vi "Create.vi"(8 "error in (no error)":errorcluster, 10 "Data Count":i32) -> (0 "error out":errorcluster, 3 "Data Count Msg out":refnum<class "Data Count Msg.lvclass">)   [LabVIEW 2022 SP3, in "Scratchpad.lvlib" / "Test 1.lvlib" / "Data Count Msg.lvclass"]
uses:
  Data Count Msg.lvclass
  Data Count Msg.lvclass/Data Count Msg.ctl
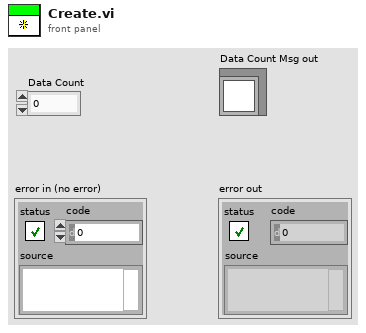
[diagram p1: front panel]
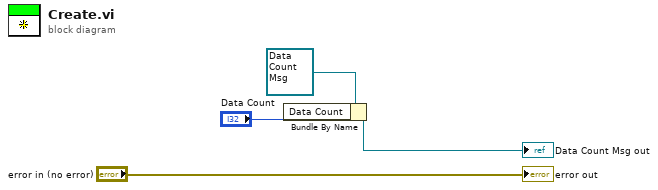
[diagram p0: block diagram]
diagram:
  n1 = Bundle By Name(cluster=refnum<class "Data Count Msg.lvclass"> refnum ("Data Count Msg in"), "Data Count"="Data Count") -> (→"Data Count Msg out":refnum<class "Data Count Msg.lvclass">)
  "error out" <- "error in (no error)"
